vi "Get_all_functions.vi"() -> (3 "Array":string[](array[string]))   [LabVIEW 2025]
uses:
  <vilib>/regexp/Match Regular Expression.xnode
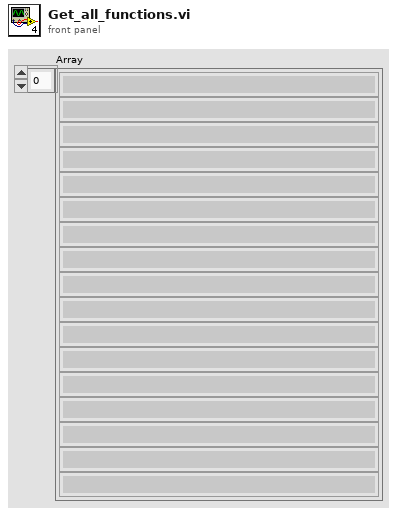
[diagram p1: front panel]
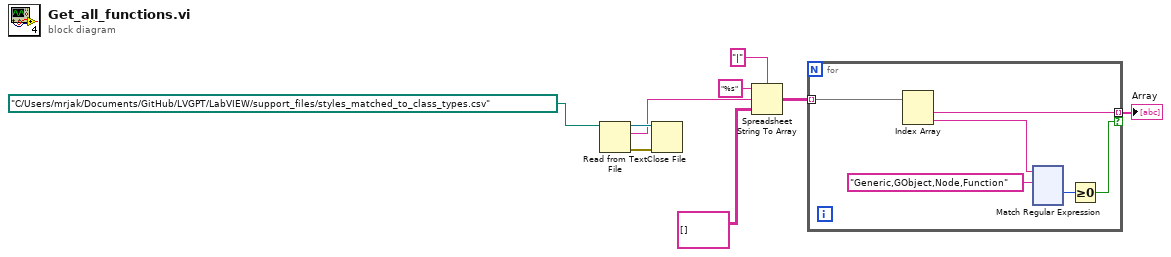
[diagram p0: block diagram]
diagram:
  n1 = Read from Text File(file (use dialog)=path "C:/Users/mrjak/Documents/GitHub/LVGPT/LabVIEW/support_files/styles_matched_to_class_types.csv") -> (refnum out=w7:refnum<file>, text=w3:string, error out=w8:errorcluster)  [unwired: 3 in, 1 out]
  n2 = Close File(refnum=w7, error in=w8) -> ()  [unwired: 2 out]
  n3 = Spreadsheet String To Array(delimiter (Tab)="|", format string="%s", spreadsheet string=w3, array type (2D Dbl)=string[][] []) -> (array=w4:string[][])
  n4 = for {
    tunnel: w4 -> [w15] mode=indexing
    tunnel: [w11] -> w1 mode=indexing if=w10
    n5 = Index Array(array=w15) -> (element #1=w11:string, element #2=w12:string)  [unwired: 2 in]
    n6 = xnode "Match Regular Expression"("input string"=w12, "regular expression"="Generic,GObject,Node,Function") -> ("offset past match"=w13:i32)  [unwired: 4 in, 4 out]
    n7 = Greater Or Equal To 0?(x=w13) -> (x >= 0?=w10:bool)
  }
  "Array" <- w1
